vi "Hide Event.vi"(8 "error in (no error)":errorcluster, 10 "Panel":string) -> (0 "error out":errorcluster)   [LabVIEW 2019, in "Panel.lvlib" / "Panel Registry.lvclass"]
doc: "Broadcasts a \"Hidden\" message to of child panels.\n\n----\nPlease see the following web address for additional documentation and tutorial information:\nhttp://www.mooregoodideas.com/mgi-panel-manager/\n\nAuthor: Derek Trepanier\n\nCopyright (c) 2018, Moore Good Ideas, Inc.\n\nAll rights reserved.\n\nRedistribution and use in source and binary forms, with or without modification, are permitted provided that the following conditions are met:\n\n * Redistributions of source code must retain the above copyright notice, this list of conditions and the following disclaimer.\n * Redistributions in binary form must reproduce the above copyright notice, this list of conditions and the following disclaimer in the documentation and/or other materials provided with the distribution.\n * Neither the name of Moore Good Ideas, Inc. nor the names of its contributors may be used to endorse or promote products derived from this software without specific prior written permission.\n\nTHIS SOFTWARE IS PROVIDED BY THE COPYRIGHT HOLDERS AND CONTRIBUTORS \"AS IS\" AND ANY EXPRESS OR IMPLIED WARRANTIES, INCLUDING, BUT NOT LIMITED TO, THE IMPLIED WARRANTIES OF MERCHANTABILITY AND FITNESS FOR A PARTICULAR PURPOSE ARE DISCLAIMED. IN NO EVENT SHALL THE COPYRIGHT OWNER OR CONTRIBUTORS BE LIABLE FOR ANY DIRECT, INDIRECT, INCIDENTAL, SPECIAL, EXEMPLARY, OR CONSEQUENTIAL DAMAGES (INCLUDING, BUT NOT LIMITED TO, PROCUREMENT OF SUBSTITUTE GOODS OR SERVICES; LOSS OF USE, DATA, OR PROFITS; OR BUSINESS INTERRUPTION) HOWEVER CAUSED AND ON ANY THEORY OF LIABILITY, WHETHER IN CONTRACT, STRICT LIABILITY, OR TORT (INCLUDING NEGLIGENCE OR OTHERWISE) ARISING IN ANY WAY OUT OF THE USE OF THIS SOFTWARE, EVEN IF ADVISED OF THE POSSIBILITY OF SUCH DAMAGE."
uses:
  Panel Registry.lvclass
  Panel Registry.lvclass/Panel Registry.ctl
  Panel Helper/Events.ctl
  Panel Helper/Panel Helper.lvclass
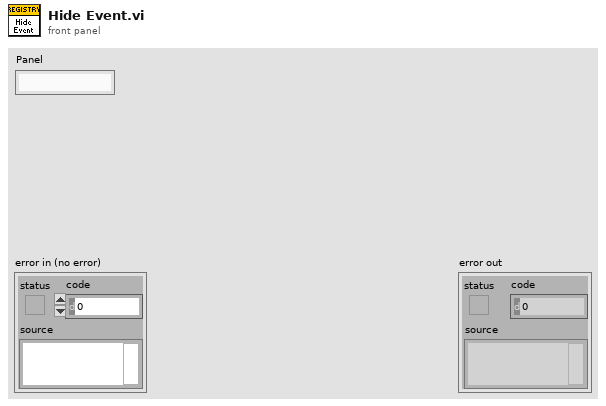
[diagram p1: front panel]
types:
  T1 = typedef "Panel.lvlib/Panel Helper.lvclass/Events.ctl" = enum16{"Initialized", "Shown", "Hidden", "Closed"}
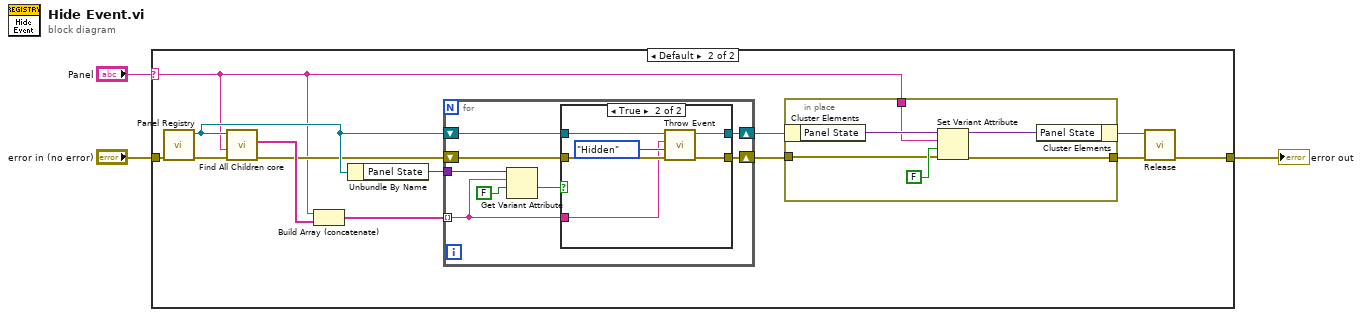
[diagram p0: block diagram]
diagram:
  n1 = case shown="Default" "Panel" {
    selector: "Panel" -> [_ w7]
    tunnel: "error in (no error)" -> [w4 w17]
    tunnel: [w4 w16] -> w2
    frame "" {
    }
    frame Default {
      n2 = call "Panel Registry.vi"("error in (no error)"=w17) -> ("error out"=w15:errorcluster, "Panel Registry out"=w11:refnum<class "Panel Registry.lvclass">)  [unwired: 9 in]
      n3 = call "Find All Children core.vi"("error in (no error)"=w15, "Panel"=w7, "Panel Registry in"=w11) -> ("error out"=w10:errorcluster, "All Children"=w14:string[])  [unwired: 7 in]
      n4 = Build Array (concatenate)(w7, w14) -> (w12:string[])
      n5 = Unbundle By Name(w11) -> ("Panel State"=w13:variant)
      n6 = for {
        shift-right: [w28] -> w8
        shift-left: w10 -> [w31]
        tunnel: w12 -> [w26] mode=indexing
        shift-right: [w30] -> w9
        shift-left: w11 -> [w29]
        tunnel: w13 -> [w27]
        n7 = Get Variant Attribute(Variant=w27, name=w26, default value (empty Variant)=FALSE) -> (value=w24:bool)  [unwired: 1 in, 3 out]
        n8 = case shown="True" w24 {
          tunnel: w31 -> [w32 w39]
          tunnel: [w33 w38] -> w30
          tunnel: w29 -> [w33 w37]
          tunnel: [w32 w36] -> w28
          tunnel: w26 -> [_ w34]
          frame False {
          }
          frame True {
            n9 = call "Throw Event.vi"("error in (no error)"=w39, "Event"=Events."Hidden", "Panel"=w34, "Panel Registry in"=w37) -> ("error out"=w36:errorcluster, "Panel Registry out"=w38:refnum<class "Panel Registry.lvclass">)  [unwired: 6 in]
          }
        }
      }
      n10 = in-place {
        in-place-border: [w22] -> w5
        in-place-border: w8 -> [w19]
        in-place-border: w7 -> [w18]
        n11 = in-place-cluster #1(w9) -> ("Panel State"=w23:variant)
        n12 = Set Variant Attribute(Variant=w23, name=w18, value=FALSE, error in=w19) -> (Variant out=w20:variant, error out=w22:errorcluster)  [unwired: 1 out]
        n13 = in-place-cluster #1("Panel State"=w20) -> (w6:refnum<class "Panel Registry.lvclass">)
      }
      n14 = call "Release.vi"("error in (no error)"=w5, "Panel Registry in"=w6) -> ("error out"=w16:errorcluster)  [unwired: 9 in]
    }
  }
  "error out" <- w2
